vi "索引1D数组(I8).vi"(8 "error in (no error)":errorcluster caption="错误输入（无错误）", 10 "索引":i32[](array[numeric]), 11 "输入数组":i8[](array[numeric])) -> (0 "error out":errorcluster caption="错误输出", 3 "元素":i8[](array[numeric]))   [LabVIEW 2012]
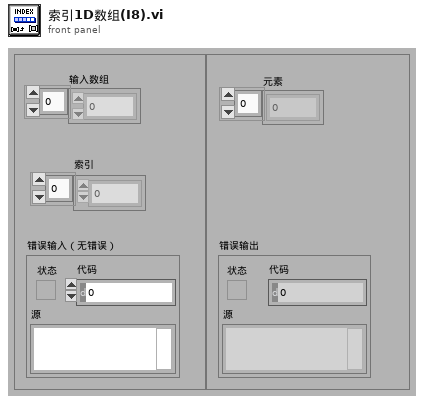
[diagram p1: front panel]
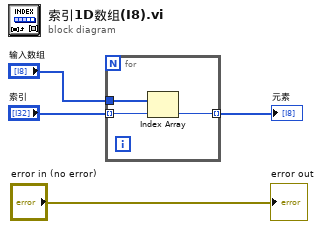
[diagram p0: block diagram]
diagram:
  n1 = for {
    tunnel: "索引" -> [w7] mode=indexing
    tunnel: "输入数组" -> [w6]
    tunnel: [w5] -> w2 mode=indexing
    n2 = Index Array(array=w6, index=w7) -> (element=w5:i8)
  }
  "元素" <- w2
  "error out" <- "error in (no error)"
